vi "FdxCmdRxVLControlEXCvi.vi"(8 "error in":errorcluster, 9 "VLControlEx":T1 {"CtrlBufInt" format="%x" items=["FDX_RX_VL_NOBI"=4096, "DX_RX_VL_BFI "=8192, "FDX_RX_VL_HFI"=12288, "FDX_RX_VL_QFI"=16384]; "CtrlBufStoreMod" items=["FDX_RX_VL_CYC"=256]; "CtrlOutStrobeGen" items=["FDX_RX_VL_NOS "=16, "FDX_RX_VL_STR"=32, "FDX_RX_VL_EST"=64]; "CtrlInt" items=["FDX_RX_VL_NOINT"=1, "FDX_RX_VL_INT"=2, "FDX_RX_VL_INT_ERR"=3]}, 11 "InstrumentHandle_port":u32) -> (0 "error out":errorcluster, 3 "InstrumentHandle_port":u32)   [LabVIEW 2020, in "AIM664LV.lvlib"]
doc: "This function is to control the extended Virtual link specific setting for a receive port. This command can only be applied if the corresponding VL has been previously setup with the AiFdxCmdRxVLControl command and the VL is operating in FDX_RX_VL_ENA_EXT mode."
uses:
  AIM664LV.lvlib
  AFDX_LibraryAdmin/FdxGlobalDllPath.vi
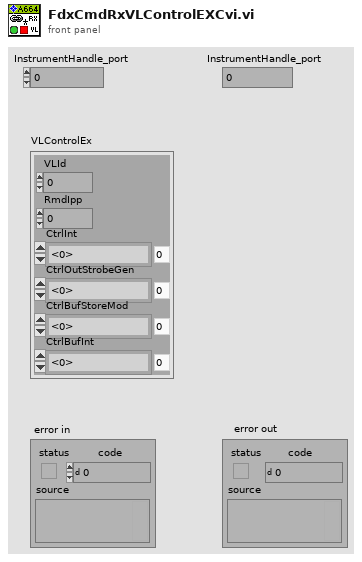
[diagram p1: front panel]
types:
  T1 = cluster{"VLId":u32, "RmdIpp":u32, "CtrlInt":u32, "CtrlOutStrobeGen":u32, "CtrlBufStoreMod":u32, "CtrlBufInt":u32}
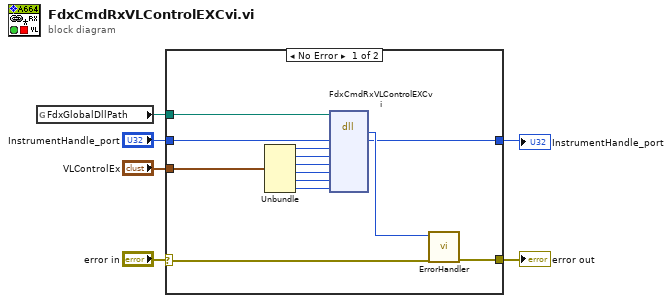
[diagram p0: block diagram]
diagram:
  n1 = global read "FdxGlobalDllPath.vi" "FdxGlobalDllPath"() -> (w4:path)
  n2 = case shown="No Error" "error in" {
    selector: "error in" -> [w18 w21]
    tunnel: [w19 w21] -> w6
    tunnel: w4 -> [w10 _]
    tunnel: [w9 w20] -> w3
    tunnel: "InstrumentHandle_port" -> [w8 w20]
    tunnel: "VLControlEx" -> [w7 _]
    frame No Error {
      n3 = Unbundle(w7) -> ("VLId"=w16:u32, "RmdIpp"=w15:u32, "CtrlInt"=w14:u32, "CtrlOutStrobeGen"=w13:u32, "CtrlBufStoreMod"=w12:u32, "CtrlBufInt"=w11:u32)
      n4 = dll-call lib="aim_fdx.19.dll" fn="FdxCmdRxVLControlEXCvi"(path in=w10, "InstrumentHandle"=w8, "VLId"=w16, "RmdIpp"=w15, "CtrlInt"=w14, "CtrlOutStrobeGen"=w13, "CtrlBufStoreMod"=w12, "CtrlBufInt"=w11) -> ("status"=w17:i32, "InstrumentHandle"=w9:u32)  [unwired: 8 in, 2 out]
      n5 = call "ErrorHandler.vi"("error in"=w18, "AIM Error"=w17) -> ("error out"=w19:errorcluster)  [unwired: 9 in]
    }
    frame Error {
    }
  }
  "error out" <- w6
  "InstrumentHandle_port" <- w3
